vi "Write temperature.vi"(8 "error in (no error)":errorcluster, 10 "temperature":dbl[](array[numeric]), 11 "ElectrometerState in":refnum<class "ElectrometerState.lvclass">) -> (0 "error out":errorcluster, 3 "ElectrometerState out":refnum<class "ElectrometerState.lvclass">)   [LabVIEW 2016, in "ElectrometerState.lvclass"]
uses:
  ElectrometerState.lvclass
  ElectrometerState.lvclass/ElectrometerState.ctl
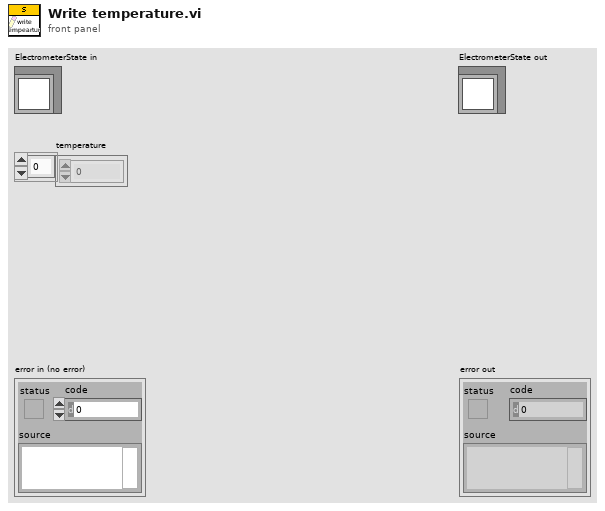
[diagram p1: front panel]
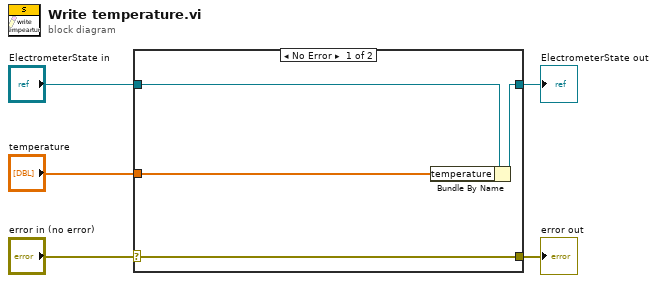
[diagram p0: block diagram]
diagram:
  n1 = case shown="No Error" "error in (no error)" {
    selector: "error in (no error)" -> [w9 w10]
    tunnel: [w9 w10] -> w4
    tunnel: [w7 w11] -> w2
    tunnel: "ElectrometerState in" -> [w8 w11]
    tunnel: "temperature" -> [w6 _]
    frame No Error {
      n2 = Bundle By Name(cluster=w8, "temperature"=w6) -> (w7:refnum<class "ElectrometerState.lvclass">)
    }
    frame Error {
    }
  }
  "error out" <- w4
  "ElectrometerState out" <- w2
